vi "Teleop.vi"(10 "Match Info":T1={"Autonomous Elapsed Seconds"=0.0, "TeleOp Elapsed Seconds"=0.0, "Disabled Elapsed Seconds"=0.0, "Visited Autonomous"=FALSE, "Visited TeleOp"=FALSE, "Visited Disabled"=FALSE, "Autonomous Settings"={"Autonomous Style"=enum."Independent", "VI Refnum"=refnum}}, 11 "Call Context":T2) -> ()   [LabVIEW 2017]
doc: "This VI is called for each TeleOp packet received from the DS where the robot is not disabled. It is often used to read from the joysticks and update I/O or to update setpoints for timed control loops. It should complete and return within 20 milliseconds or it may miss DS packets."
uses:
  <vilib>/Rock Robotics/WPI/DriverStation/WPI_DriverStationDerivedRobotMode.ctl
  <vilib>/Rock Robotics/WPI/DriverStation/WPI_DriverStationMatch Info.ctl
  <vilib>/Rock Robotics/WPI/ThirdParty/Phoenix-LabVIEW/Motor Controller/Controls/CTRE_Phoenix_MotorControl_ControlMode.ctl
  <vilib>/Rock Robotics/WPI/ThirdParty/Sensors/navX/_TypeDefs/Flags/Z900_navX_Flags_OpStatusTypeDef.ctl
  <vilib>/Rock Robotics/WPI/Utilities/WPI_GetSetVariantRefNum.vi
  <vilib>/Rock Robotics/Network Tables/NT Write Boolean Array.vi
  <vilib>/Rock Robotics/Network Tables/NT Write Numeric Array.vi
  <vilib>/Rock Robotics/Network Tables/NT Read Boolean.vi
  <vilib>/Rock Robotics/Network Tables/NT Read Number.vi
  <vilib>/Rock Robotics/WPI/ThirdParty/Phoenix-LabVIEW/Pigeon IMU/CTRE_PigeonIMU_GetTempStateUpTime.vi
  <vilib>/Rock Robotics/WPI/ThirdParty/Phoenix-LabVIEW/Pigeon IMU/CTRE_PigeonIMU_GetFusedHeading.vi
  <vilib>/Rock Robotics/WPI/ThirdParty/Phoenix-LabVIEW/Pigeon IMU/CTRE_PigeonIMU_GetYPR.vi
panel:
  in  "Self Righting":bool
  out "lift":dbl
  in  "D Gain":dbl=0.0004 format="%#_13g"
  in  "P Gain":dbl=0.04 format="%#_13g"
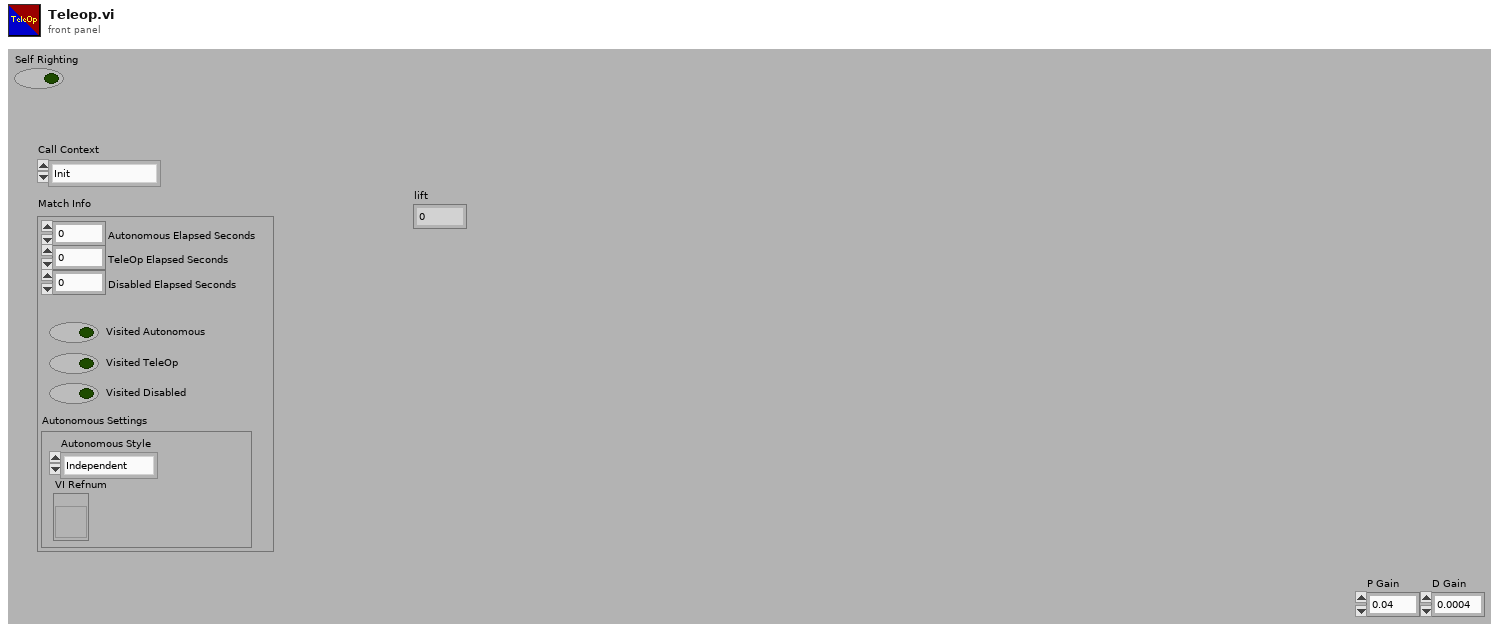
[diagram p1: front panel]
types:
  T1 = typedef "WPI_DriverStationMatch Info.ctl" = cluster{"Autonomous Elapsed Seconds":dbl, "TeleOp Elapsed Seconds":dbl, "Disabled Elapsed Seconds":dbl, "Visited Autonomous":bool, "Visited TeleOp":bool, "Visited Disabled":bool, "Autonomous Settings":cluster{"Autonomous Style":enum16{"Iterative", "Independent"}, "VI Refnum":refnum<vi>}}
  T2 = typedef "WPI_DriverStationDerivedRobotMode.ctl" = enum16{"Init", "Execute", "Stop"}
  T3 = typedef "CTRE_Phoenix_MotorControl_ControlMode.ctl" = u16
  T4 = typedef "WPI_JoystickDevRef.ctl" = cluster{"Device":T5}
  T5 = typedef "WPI_JoystickDeviceEnum.ctl" = enum16{"USB 0", "USB 1", "USB 2", "USB 3", "USB 4", "USB 5"}
  T6 = typedef "WPI_MotorControlDeviceRef.ctl" = cluster{"DeviceStatus":errorcluster, "Type":T7, "PWM":cluster{"PWM Channel":T8, "DeadBand":T9}, "CAN":cluster{"Device Number":u8, "SetOutput VI Ref":variant, "GetOutput VI Ref":variant, "Enable VI Ref":variant, "Disable VI Ref":variant, "Data":variant}, "Invert":bool, "DIO PWM":cluster{"PWM \"Enable\" Channel":T8, "DIOChannel":T10, "PWM Rate":dbl}}
  T7 = typedef "WPI_MotorControlType.ctl" = enum16{"PWM", "CAN", "DIO PWM"}
  T8 = typedef "FPGA_DIOPWMChannel.ctl" = enum8{"PWM 0", "PWM 1", "PWM 2", "PWM 3", "PWM 4", "PWM 5", "PWM 6", "PWM 7", "PWM 8", "PWM 9", "PWM MXP 0", "PWM MXP 1", "PWM MXP 2", "PWM MXP 3", "PWM MXP 4", "PWM MXP 5", "PWM MXP 6", "PWM MXP 7", "PWM MXP 8", "PWM MXP 9", "Invalid"}
  T9 = typedef "WPI_PWMDeadband.ctl" = cluster{"Name":string, "maxPositivePwm":i32, "minPositivePwm":i32, "centerPwm":i32, "maxNegativePwm":i32, "minNegativePwm":i32, "angularRange":u16}
  T10 = typedef "FPGA_DIOChannel.ctl" = enum8{"DIO 0", "DIO 1", "DIO 2", "DIO 3", "DIO 4", "DIO 5", "DIO 6", "DIO 7", "DIO 8", "DIO 9", "DIO MXP 0", "DIO MXP 1", "DIO MXP 2", "DIO MXP 3", "DIO MXP 4", "DIO MXP 5", "DIO MXP 6", "DIO MXP 7", "DIO MXP 8", "DIO MXP 9", "DIO MXP 10", "DIO MXP 11", "DIO MXP 12", "DIO MXP 13", "DIO MXP 14", "DIO MXP 15", "SPI Port CS1", "SPI Port CS2", "SPI Port CS3", "SPI Port MISO", "SPI Port MOSI", "Invalid"}
  T11 = typedef "CTRE_PigeonIMU_DeviceRef.ctl" = cluster{"DeviceStatus":errorcluster, "Device Number":u8, "Type":T12, "Device ID":u32, "Handle":u64, "UsageFrame":u32, "Library Path":path}
  T12 = typedef "CTRE_PigeonIMU_ConnectionType.ctl" = u32
  T13 = typedef "CTRE_PigeonIMU_CalibrationMode.ctl" = u16
  T14 = typedef "CTRE_PigeonIMU_PigeonState.ctl" = enum16{"NoComm", "Initializing", "Ready", "UserCalibration"}
  T15 = cluster{"CurrentMode":T13, "LastCalError":i32, "CalBooting?":bool, "PigeonState":T14, "UpTime":u32, "Temp. (C)":dbl, "Temp Compensation Event Count":u32, "No Motion Event Count":u32}
  T16 = cluster{"Heading":dbl, "Valid?":bool, "Fusing?":bool}
  T17 = typedef "Z900_navX_Flags_OpStatusTypeDef.ctl" = u8
  T18 = typedef "WPI_RobotDriveDevRef.ctl" = cluster{"DevStatus":errorcluster, "Motors[]":T6[], "Square Inputs":bool, "Max Output":dbl}
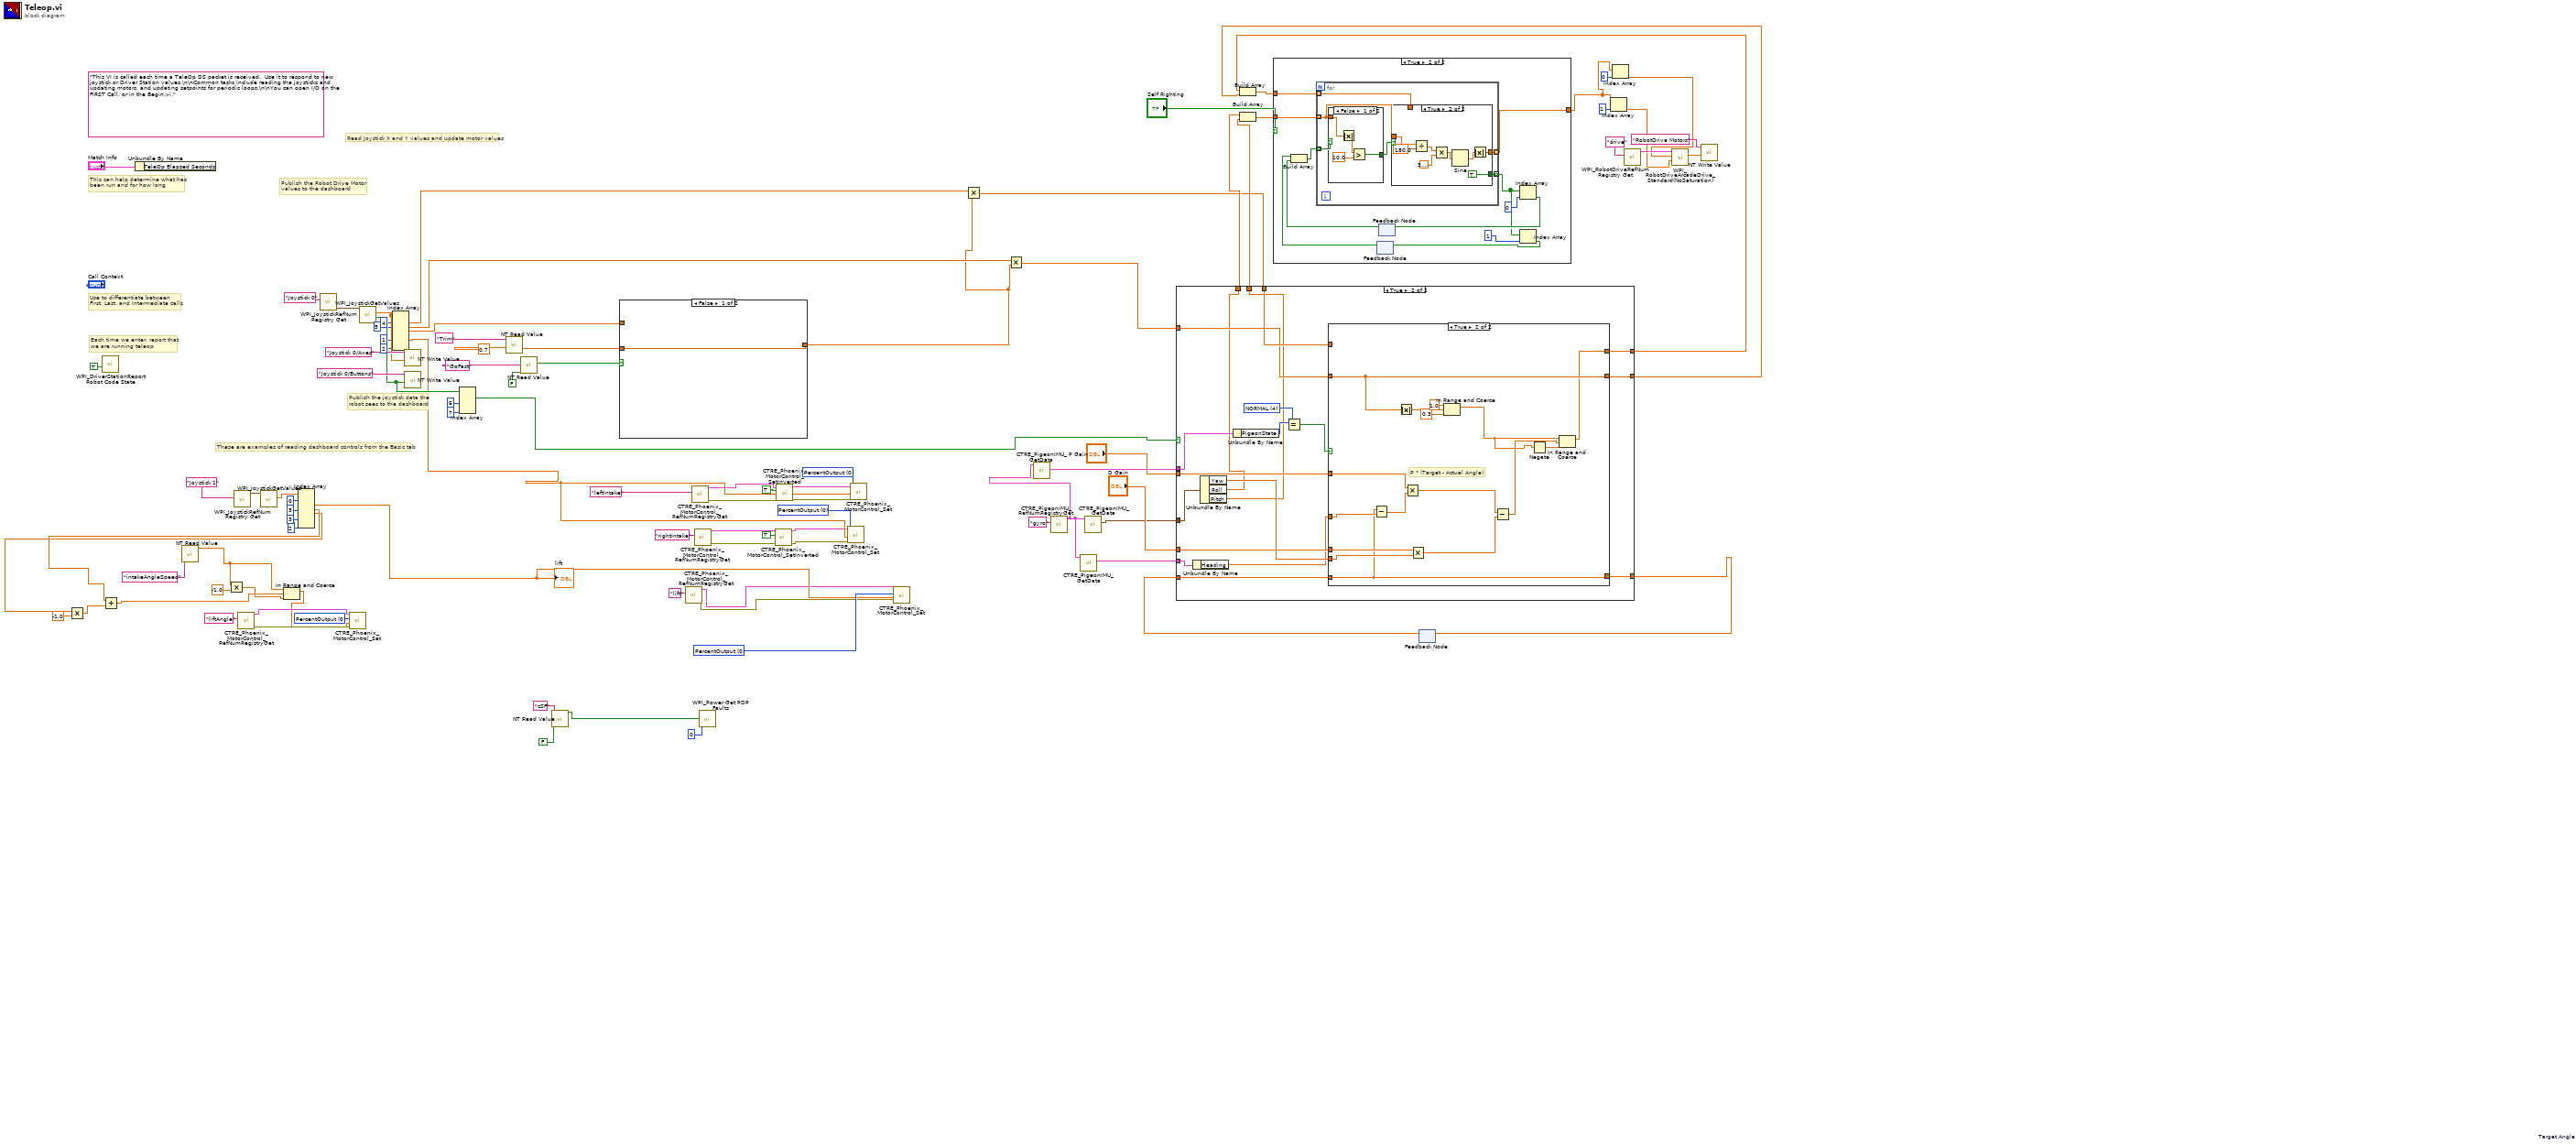
[diagram p0: block diagram]
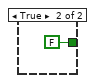
[diagram p4: hidden frame]
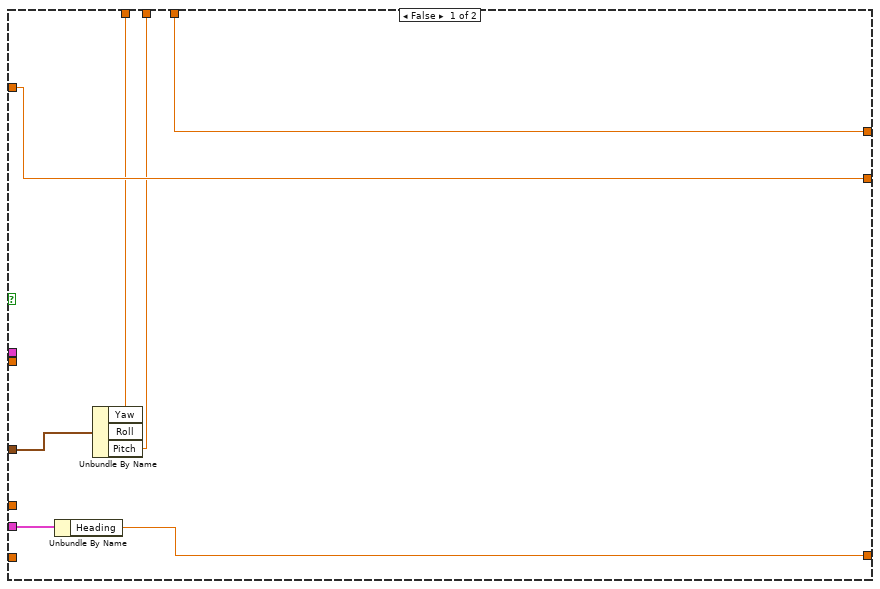
[diagram p5: hidden frame]
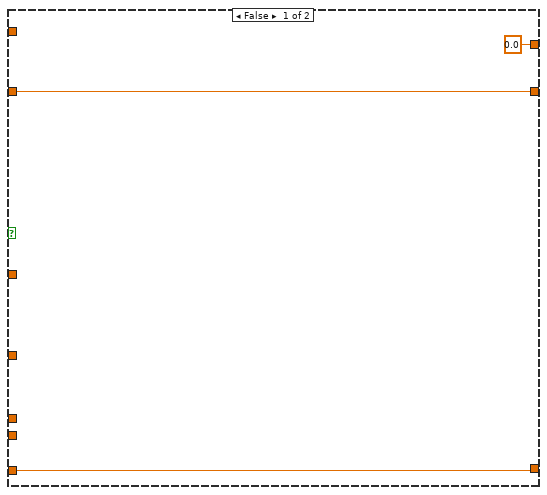
[diagram p6: hidden frame]
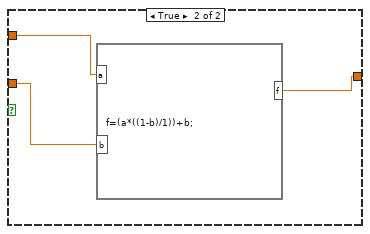
[diagram p7: hidden frame]
diagram:
  w40 = T3 0 items=["PercentOutput"=0, "Position"=1, "Velocity"=2, "Current"=3, "Follower"=5, "MotionProfile"=6, "MotionMagic"=7, "MotionMagicArc"=8, "MotionProfileArc"=10, "Disabled"=15] ("Control Mode")
  w42 = T3 0 items=["PercentOutput"=0, "Position"=1, "Velocity"=2, "Current"=3, "Follower"=5, "MotionProfile"=6, "MotionMagic"=7, "MotionMagicArc"=8, "MotionProfileArc"=10, "Disabled"=15] ("Control Mode")
  w43 = T3 0 items=["PercentOutput"=0, "Position"=1, "Velocity"=2, "Current"=3, "Follower"=5, "MotionProfile"=6, "MotionMagic"=7, "MotionMagicArc"=8, "MotionProfileArc"=10, "Disabled"=15] ("Control Mode")
  w53 = T3 0 items=["PercentOutput"=0, "Position"=1, "Velocity"=2, "Current"=3, "Follower"=5, "MotionProfile"=6, "MotionMagic"=7, "MotionMagicArc"=8, "MotionProfileArc"=10, "Disabled"=15] ("Control Mode")
  (unwired) "This VI is called each time a TeleOp DS packet is received.  Use it to respond to new joystick or Driver Station values.\n\nCommon tasks include reading the joysticks and updating motors, and updating setpoints for periodic loops.\n\nYou can open I/O on the FIRST Call, or in the Begin.vi."
  # "These are examples of reading dashboard controls from the Basic tab"
  # "Publish the Robot Drive Motor\nvalues to the dashboard"
  # "Publish the joystick data the\nrobot sees to the dashboard"
  # "Each time we enter, report that\nwe are running teleop"
  # "Use to differentiate between\nFirst, Last, and Intermediate calls"
  # "This can help determine what has\nbeen run and for how long"
  # "Read Joystick X and Y values and update motor values"
  n1 = call <vilib>:"WPI_DriverStationReport Robot Code State.vi"("TeleOp"=TRUE ("Autonomous")) -> ()  [unwired: 10 in, 1 out]
  n2 = Unbundle By Name("Match Info") -> ()  [unwired: 1 out]
  n3 = call-poly <vilib>:"NT Read Value.vi"("Name"="intakeAngleSpeed") -> ("Numeric"=w32:dbl)  [unwired: 9 in, 1 out]
  n4 = Multiply(x=w32, y=-1.0) -> (x*y=w30:dbl)
  n5 = call <vilib>:"WPI_JoystickRefNum Registry Get.vi"("refnum name"="Joystick 1") -> ("JoystickDevRef"=w49:T4)  [unwired: 1 in, 9 out]
  n6 = call <vilib>:"CTRE_Phoenix_MotorControl_RefNumRegistryGet.vi"("refnum name"="liftAngle") -> ("error out"=w35:errorcluster, "PhoenixMotorControlDevRef"=w36:T6)  [unwired: 9 in]
  n7 = call <vilib>:"WPI_JoystickGetValues.vi"("JoystickDevRef"=w49) -> ("Axes"=w48:dbl[])  [unwired: 6 in, 4 out]
  n8 = Index Array(array=w48, index #1=0 ("index"), index #2=5 ("index"), index #3=3 ("index"), index #4=2 ("index")) -> (element #2=w38:dbl, element #3=w13:dbl, element #4=w12:dbl)  [unwired: 3 in, 4 out]
  "lift" <- w38
  n9 = Multiply(x=w12, y=-1.0) -> (x*y=w10:dbl)
  n10 = Add(x=w13, y=w10) -> (x+y=w9:dbl)
  n11 = In Range and Coerce(upper limit=w32, x=w9, lower limit=w30) -> (coerced(x)=w34:dbl)  [unwired: 1 out]
  n12 = call <vilib>:"WPI_JoystickRefNum Registry Get.vi"("refnum name"="Joystick 0") -> ("JoystickDevRef"=w93:T4)  [unwired: 1 in, 9 out]
  n13 = call <vilib>:"CTRE_Phoenix_MotorControl_Set.vi"("error in (no error)"=w35, "Output"=w34, "Control Mode"=w40, "PhoenixMotorControlDevRef"=w36) -> ()  [unwired: 6 in, 2 out]
  n14 = call <vilib>:"WPI_JoystickGetValues.vi"("JoystickDevRef"=w93) -> ("Buttons"=w73:bool[], "Axes"=w89:dbl[])  [unwired: 6 in, 3 out]
  n15 = Index Array(array=w89, index #1=4 ("index"), index #2=5 ("index"), index #3=2 ("index"), index #5=1 ("index")) -> (element #1=w78:dbl, element #2=w80:dbl, element #3=w69:dbl, element #5=w68:dbl)  [unwired: 3 in, 3 out]
  n16 = call-poly <vilib>:"NT Write Value.vi"("Numeric Array"=w89, "Name"="Joystick 0/Axes") -> ()  [unwired: 9 in, 1 out]
  n17 = call-poly <vilib>:"NT Write Value.vi"("Boolean Array"=w73, "Name"="Joystick 0/Buttons") -> ()  [unwired: 9 in, 1 out]
  n18 = Index Array(array=w73, index #2=6 ("index"), index #3=7 ("index")) -> (element #1=w72:bool)  [unwired: 2 in, 3 out]
  n19 = call-poly <vilib>:"NT Read Value.vi"("Default Value"=0.7, "Name"="Trim" ("refnum name")) -> ("Numeric"=w81:dbl)  [unwired: 8 in, 1 out]
  n20 = call-poly <vilib>:"NT Read Value.vi"("Default Value"=FALSE, "Name"="GoFast" ("refnum name")) -> ("Boolean"=w82:bool)  [unwired: 8 in, 1 out]
  n21 = call-poly <vilib>:"NT Read Value.vi"("Default Value"=FALSE, "Name"="cSF") -> ("Boolean"=w27:bool)  [unwired: 8 in, 1 out]
  n22 = case shown="False" w82 {
    tunnel: [w98 w101] -> w79
    tunnel: w81 -> [w98 w100]
    tunnel: w69 -> [_ w99]
    frame False {
    }
    frame True {
      n23 = formula code="f=(a*((1-b)/1))+b;"("a"=w99, "b"=w100) -> ("f"=w101:dbl)
    }
  }
  n24 = call <vilib>:"CTRE_Phoenix_MotorControl_RefNumRegistryGet.vi"("refnum name"="lift") -> ("error out"=w29:errorcluster, "PhoenixMotorControlDevRef"=w28:T6)  [unwired: 9 in]
  n25 = call <vilib>:"CTRE_Phoenix_MotorControl_RefNumRegistryGet.vi"("refnum name"="leftIntake") -> ("error out"=w22:errorcluster, "PhoenixMotorControlDevRef"=w23:T6)  [unwired: 9 in]
  n26 = call <vilib>:"CTRE_Phoenix_MotorControl_RefNumRegistryGet.vi"("refnum name"="rightIntake") -> ("error out"=w18:errorcluster, "PhoenixMotorControlDevRef"=w19:T6)  [unwired: 9 in]
  n27 = call <vilib>:"WPI_Power Get PDP Faults.vi"("Power Distribution Panel (0)"=u8 0, "Clear Sticky Faults"=w27) -> ()  [unwired: 9 in, 5 out]
  n28 = call <vilib>:"CTRE_Phoenix_MotorControl_SetInverted.vi"("error in (no error)"=w18, "Invert?"=TRUE, "PhoenixMotorControlDevRef"=w19) -> ("error out"=w16:errorcluster, "PhoenixMotorControlDevRef"=w17:T6)  [unwired: 7 in]
  n29 = call <vilib>:"CTRE_Phoenix_MotorControl_SetInverted.vi"("error in (no error)"=w22, "Invert?"=TRUE, "PhoenixMotorControlDevRef"=w23) -> ("error out"=w20:errorcluster, "PhoenixMotorControlDevRef"=w21:T6)  [unwired: 7 in]
  n30 = call <vilib>:"CTRE_Phoenix_MotorControl_Set.vi"("error in (no error)"=w16, "Output"=w68, "Control Mode"=w43, "PhoenixMotorControlDevRef"=w17) -> ()  [unwired: 6 in, 2 out]
  n31 = call <vilib>:"CTRE_Phoenix_MotorControl_Set.vi"("error in (no error)"=w20, "Output"=w68, "Control Mode"=w42, "PhoenixMotorControlDevRef"=w21) -> ()  [unwired: 6 in, 2 out]
  n32 = call <vilib>:"CTRE_Phoenix_MotorControl_Set.vi"("error in (no error)"=w29, "Output"=w38, "Control Mode"=w53, "PhoenixMotorControlDevRef"=w28) -> ()  [unwired: 6 in, 2 out]
  n33 = Multiply(x=w78, y=w79) -> (x*y=w58:dbl)
  n34 = Multiply(x=w80, y=w79) -> (x*y=w62:dbl)
  n35 = call <vilib>:"CTRE_PigeonIMU_RefNumRegistryGet.vi"("refnum name"="gyro") -> ("PigeonIMUDevRef"=w4:T11)  [unwired: 9 in, 1 out]
  n36 = call-poly <vilib>:"CTRE_PigeonIMU_GetData.vi"("PigeonIMUDevRef"=w4) -> ("Temp/State/UpTime"=w5:T15)  [unwired: 8 in, 2 out]
  n37 = call-poly <vilib>:"CTRE_PigeonIMU_GetData.vi"("PigeonIMUDevRef"=w4) -> ("Fused Heading"=w6:T16)  [unwired: 8 in, 2 out]
  n38 = call-poly <vilib>:"CTRE_PigeonIMU_GetData.vi"("PigeonIMUDevRef"=w4) -> ("Yaw Pitch Roll"=w7:cluster{"Yaw":dbl, "Pitch":dbl, "Roll":dbl})  [unwired: 8 in, 2 out]
  n39 = feedback #1 "Target Angle"() -> (w75:dbl)  [unwired: 1 in]
  n40 = case shown="True" w72 {
    tunnel: "P Gain" -> [_ w123]
    tunnel: "D Gain" -> [_ w122]
    tunnel: w75 -> [_ w121]
    tunnel: w58 -> [w108 w120]
    tunnel: w62 -> [w107 w119]
    tunnel: [w107 w118] -> w56
    tunnel: [w108 w117] -> w57
    tunnel: [w102 w116] -> w74
    tunnel: [w106 w109] -> w61
    tunnel: [w105 w110] -> w60
    tunnel: w7 -> [w104 w113]
    tunnel: w6 -> [w103 w112]
    tunnel: w5 -> [_ w115]
    frame False {
      n41 = Unbundle By Name(w103) -> ("Heading"=w102:dbl)
      n42 = Unbundle By Name(w104) -> ("Roll"=w106:dbl, "Pitch"=w105:dbl)  [unwired: 1 out]
    }
    frame True {
      w126 = T17 4 items=["INITIALIZING", "SELFTEST_IN_PROGRESS", "ERROR", "IMU_AUTOCAL_IN_PROGRESS", "NORMAL"] ("y")
      n43 = Unbundle By Name(w112) -> ("Heading"=w111:dbl)
      n44 = Unbundle By Name(w113) -> ("Yaw"=w124:dbl, "Roll"=w109:dbl, "Pitch"=w110:dbl)
      n45 = Unbundle By Name(w115) -> ("PigeonState"=w114:T14)
      n46 = Equal?(x=w114, y=w126) -> (x = y?=w125:bool)
      n47 = case shown="True" w125 {
        tunnel: w111 -> [_ w145]
        tunnel: w124 -> [_ w142]
        tunnel: w123 -> [_ w143]
        tunnel: w122 -> [_ w141]
        tunnel: w121 -> [w129 w130]
        tunnel: w120 -> [_ _]
        tunnel: w119 -> [w128 w138]
        tunnel: [w128 w138] -> w118
        tunnel: [0.0 ("upper limit") w131] -> w117
        tunnel: [w129 w130] -> w116
        frame False {
        }
        frame True {
          # "P * (Target - Actual Angle)"
          n48 = Subtract(x=w130, y=w145) -> (x-y=w144:dbl)
          n49 = Absolute Value(x=w138) -> (abs(x)=w137:dbl)
          n50 = Multiply(x=w143, y=w144) -> (x*y=w140:dbl)
          n51 = Multiply(x=w141, y=w142) -> (x*y=w139:dbl)
          n52 = In Range and Coerce(upper limit=1.0, x=w137, lower limit=0.3) -> (coerced(x)=w132:dbl)  [unwired: 1 out]
          n53 = Subtract(x=w140, y=w139) -> (x-y=w134:dbl)
          n54 = Negate(x=w132) -> (-x=w133:dbl)
          n55 = In Range and Coerce(upper limit=w132, x=w134, lower limit=w133) -> (coerced(x)=w131:dbl)  [unwired: 1 out]
        }
      }
    }
  }
  n56 = Build Array(w57, w56) -> (w63:dbl[])
  n57 = Build Array(w61, w60) -> (w59:dbl[])
  n58 = case shown="True" "Self Righting" {
    tunnel: [w146 w157] -> w64
    tunnel: w63 -> [w146 w156]
    tunnel: w59 -> [_ w155]
    frame False {
    }
    frame True {
      n59 = feedback #2() -> (w150:bool)  [unwired: 1 in]
      n60 = feedback #3() -> (w151:bool)  [unwired: 1 in]
      n61 = Build Array(w150, w151) -> (w152:bool[])
      n62 = for {
        tunnel: [w163] -> w157 mode=indexing
        tunnel: w156 -> [w162] mode=indexing
        tunnel: w155 -> [w161] mode=indexing
        tunnel: [w160] -> w147 mode=indexing
        tunnel: w152 -> [w158] mode=indexing
        n63 = case shown="False" w158 {
          tunnel: w161 -> [w176 _]
          tunnel: [w174 FALSE] -> w159
          frame False {
            n64 = Absolute Value(x=w176) -> (abs(x)=w177:dbl)
            n65 = Greater?(x=w177, y=10.0) -> (0:w174:bool)
          }
          frame True {
          }
        }
        n66 = case shown="True" w159 {
          selector: w159 -> [w164 _]
          tunnel: [w165 w170] -> w163
          tunnel: w162 -> [w165 _]
          tunnel: w161 -> [_ w169]
          tunnel: [w164 TRUE] -> w160
          frame False {
          }
          frame True {
            n67 = Divide(x=w169, y=180.0) -> (x/y=w173:dbl)
            n68 = Multiply(x=w173, y=3.141592653589793) -> (x*y=w172:dbl)
            n69 = Sine(x=w172) -> (sin(x)=w171:dbl)
            n70 = Absolute Value(x=w171) -> (abs(x)=w170:dbl)
          }
        }
      }
      n71 = Index Array(array=w147, index=1) -> (element=w149:bool)
      n72 = feedback-in #2(w149) -> ()
      n73 = Index Array(array=w147, index=0) -> (element=w148:bool)
      n74 = feedback-in #3(w148) -> ()
    }
  }
  n75 = feedback-in #1(w74) -> ()
  n76 = Index Array(array=w64, index=1) -> (element=w55:dbl)
  n77 = Index Array(array=w64, index=0) -> (element=w54:dbl)
  n78 = call <vilib>:"WPI_RobotDriveRefNum Registry Get.vi"("refnum name"="drive") -> ("RobotDriveDevRef"=w95:T18)  [unwired: 1 in, 9 out]
  n79 = call <vilib>:"WPI_RobotDriveArcadeDrive_Standard(NoSaturation).vi"("Y axis value"=w55, "X axis value"=w54, "RobotDriveDevRef"=w95) -> ("Motor Values"=w88:dbl[])  [unwired: 1 in, 7 out]
  n80 = call-poly <vilib>:"NT Write Value.vi"("Numeric Array"=w88, "Name"="RobotDrive Motors") -> ()  [unwired: 9 in, 1 out]
